vi "Mean between Cursers- Plugin Main.vi"(11 "Shared Data from EMA":T2={"Impulse Positions"=[], "Parameter Impuls Series"=[], "Data File"={"Data Channels"=[], "Sample Rate"=0, "Channel List"=[]}, "desacc "={"Threshold 1 [Acc]"=7000.0, "Threshold 2 [% of TH1]"=60, "tolerance"=3, "Search WD "=0.1, " always use TH2"=FALSE, "Range"=2.0, "Max time"=120.0, "Min time"=20.0, "Velocity Threshold"=150}, "Experiment Parameters 2"={"Subject"="", "Strain"="", "Rotation plane"="", "Experimenter"="", "Trial"=0.0, "Time"=0.0}} {"Parameter Impuls Series"."Gain" format="%.1f"; "Parameter Impuls Series"."Offset" format="%.1f"}) -> (3 "Shared Data from EMA 2":T2={"Impulse Positions"=[], "Parameter Impuls Series"=[], "Data File"={"Data Channels"=[], "Sample Rate"=0, "Channel List"=[]}, "desacc "={"Threshold 1 [Acc]"=7000.0, "Threshold 2 [% of TH1]"=60, "tolerance"=3, "Search WD "=0.1, " always use TH2"=FALSE, "Range"=2.0, "Max time"=120.0, "Min time"=20.0, "Velocity Threshold"=150}, "Experiment Parameters 2"={"Subject"="", "Strain"="", "Rotation plane"="", "Experimenter"="", "Trial"=0.0, "Time"=0.0}} {"Parameter Impuls Series"."Gain" format="%.1f"; "Parameter Impuls Series"."Offset" format="%.1f"})   [LabVIEW 2013]
uses:
  Plugin Shared Data.ctl
  core/type-defs/TD_Impulse Parameter.ctl
  res/controls/impuls graph/impuls graph.xctl
  <vilib>/Analysis/baseanly.llb/Mean (DBL).vi
  comm/impulse/impulse functions.lvlib
  <vilib>/Analysis/NI_AALBase.lvlib
  <vilib>/ptbypt/NI_PtbyPt.lvlib
  core/core.lvlib
  plugin data.lvlib
panel:
  out "Waveform Graph":dbl[][](graph)
  out "Impulse Plot":T1(xcontrol)
  in  "Delete trace":bool
  in  "Button toClipboard":bool
  in  "Button Save":bool
  in  "Table":string[][](table)
  out "Mean 1":dbl format="%#.3f"
  out "Mean 2":dbl format="%#.3f"
  out "Mean 2 SD":dbl format="%#.3f"
  in  "Button Calculate":bool
  out "Mean 1 SD":dbl format="%#.3f"
  in  "Parameter Impuls Series":T3=[{"Color"=4652800, "Visible"=TRUE, "Channel"=5, "Invert"=FALSE, "Desaccade"=FALSE, "Offset"=0.0, "Gain"=1.0}, {"Color"=16860, "Visible"=TRUE, "Channel"=13, "Invert"=FALSE, "Desaccade"=FALSE, "Offset"=0.0, "Gain"=1.0}, {"Color"=16711680, "Visible"=TRUE, "Channel"=21, "Invert"=FALSE, "Desaccade"=FALSE, "Offset"=0.0, "Gain"=1.0}] {"Gain" format="%.1f"; "Offset" format="%.1f"}
  in  "Impulse Direction":bool
  in  "Mean and STD":bool
  in  "Delete trace 2":bool
  in  "Stop Button":bool
  # "Offset         Gain    Inv                    Channel                         Col   Vis   Sac"
  # "Pos"
  # "Neg"
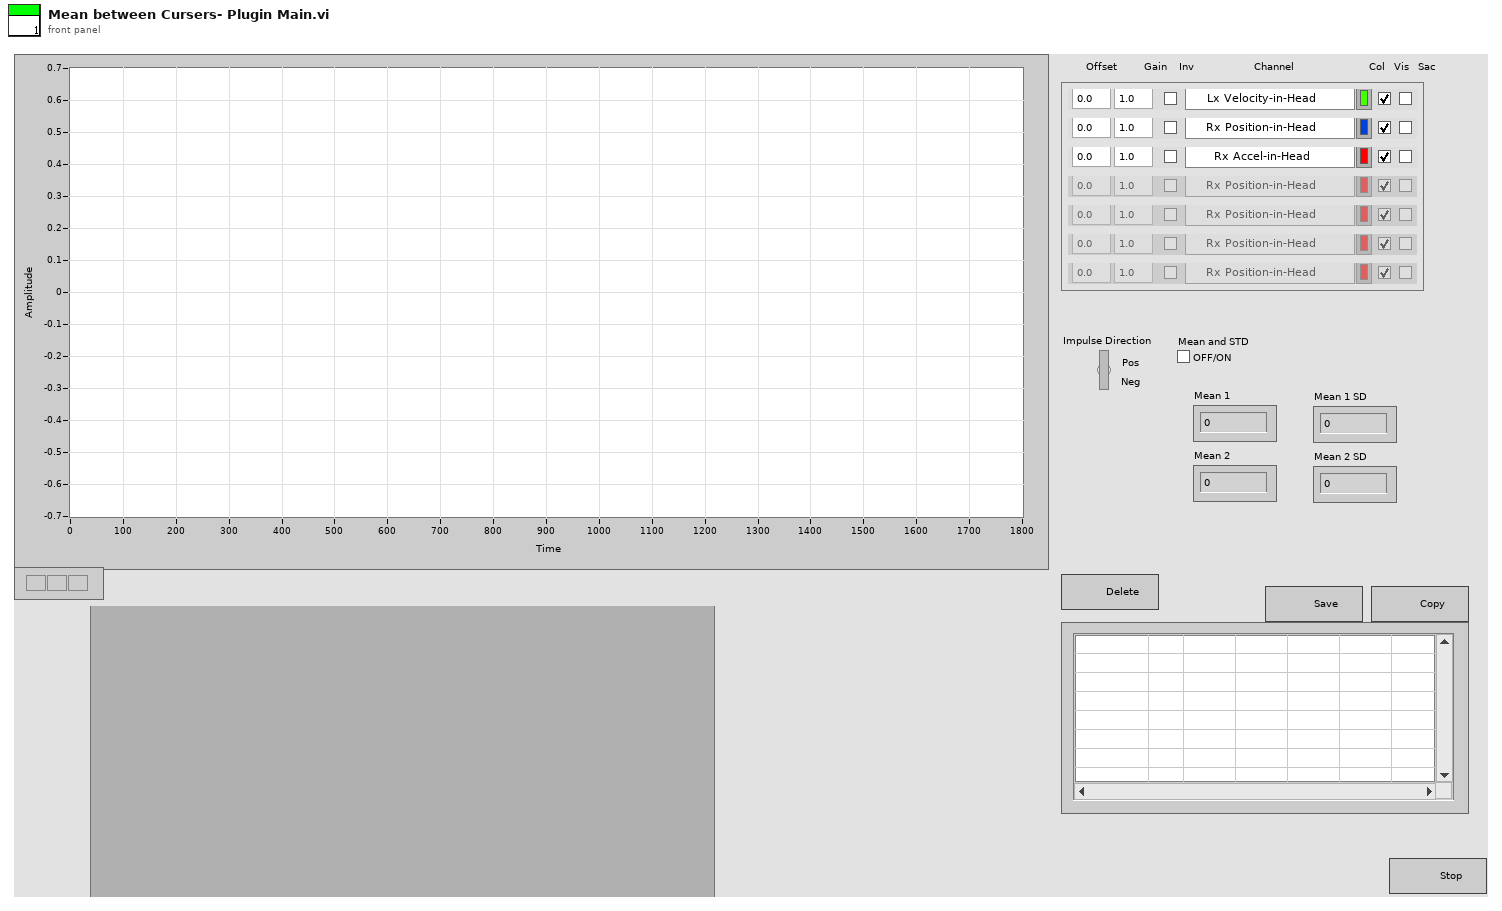
[diagram p1: front panel]
types:
  T1 = cluster{"Data":dbl[][], "Colour":u32, "Channel Name":string, "Sample Rate":dbl, "Visible":bool}[]
  T2 = typedef "plugin data.lvlib/Plugin Shared Data.ctl" = cluster{"Impulse Positions":cluster{"Start":i32, "End":i32, "Impulse Plane":enum16{"Other", "Yaw", "Pitch", "Roll", "LARP", "RALP"}, "Impulse Direction +ve?":bool, "Time offset":i32, "Amplitude offset":dbl}[], "Parameter Impuls Series":T3, "Data File":cluster{"Data Channels":dbl[][], "Sample Rate":i32, "Channel List":string[]}, "desacc ":cluster{"Threshold 1 [Acc]":dbl, "Threshold 2 [% of TH1]":i32, "tolerance":i32, "Search WD ":dbl, " always use TH2":bool, "Range":dbl, "Max time":dbl, "Min time":dbl, "Velocity Threshold":i32}, "Experiment Parameters 2":cluster{"Subject":string, "Strain":string, "Rotation plane":string, "Experimenter":string, "Trial":dbl, "Time":dbl}}
  T3 = typedef "core.lvlib/TD_Impulse Parameter.ctl" = cluster{"Color":u32, "Visible":bool, "Channel":u16, "Invert":bool, "Desaccade":bool, "Offset":dbl, "Gain":dbl}[]
  T4 = cluster{"Example Data":bool, "Impuls Data":cluster{"Data":dbl[][], "Colour":u32, "Channel Name":string, "Sample Rate":dbl, "Visible":bool}[], "K":dbl[], "cum pos data":dbl[][]}
  T5 = enum16{"Other", "Yaw", "Pitch", "Roll", "LARP", "RALP"}
  T6 = cluster{"Data Channels":dbl[][], "Sample Rate":i32, "Channel List":string[]}
  T7 = cluster{"Start":i32, "End":i32, "Impulse Plane":enum16{"Other", "Yaw", "Pitch", "Roll", "LARP", "RALP"}, "Impulse Direction +ve?":bool, "Time offset":i32, "Amplitude offset":dbl}[]
  T8 = cluster{"Threshold 1 [Acc]":dbl, "Threshold 2 [% of TH1]":i32, "tolerance":i32, "Search WD ":dbl, " always use TH2":bool, "Range":dbl, "Max time":dbl, "Min time":dbl, "Velocity Threshold":i32}
  T9 = typedef "LVCursorListTypeDef.ctl" = cluster{"Name":string, "Color":u32, "Style":u8, "Point Style":u8, "Name Visible":bool, "Allow Drag":bool, "Cursor Mode":u32, "Plot":i32, "Index":i32, "Position":cluster{"X":dbl, "Y":dbl}, "X Scale":u32, "Y Scale":u32, "Watch Plots":i32[], "Watch All Plots":bool, "Plot Area":i32, "Label Offset":cluster{"X":dbl, "Y":dbl}}[]
  T10 = cluster{"Name":string, "Color":u32, "Style":u8, "Point Style":u8, "Name Visible":bool, "Allow Drag":bool, "Cursor Mode":u32, "Plot":i32, "Index":i32, "Position":cluster{"X":dbl, "Y":dbl}, "X Scale":u32, "Y Scale":u32, "Watch Plots":i32[], "Watch All Plots":bool, "Plot Area":i32, "Label Offset":cluster{"X":dbl, "Y":dbl}}
  T11 = cluster{"Data":dbl[][], "Colour":u32, "Channel Name":string, "Sample Rate":dbl, "Visible":bool}
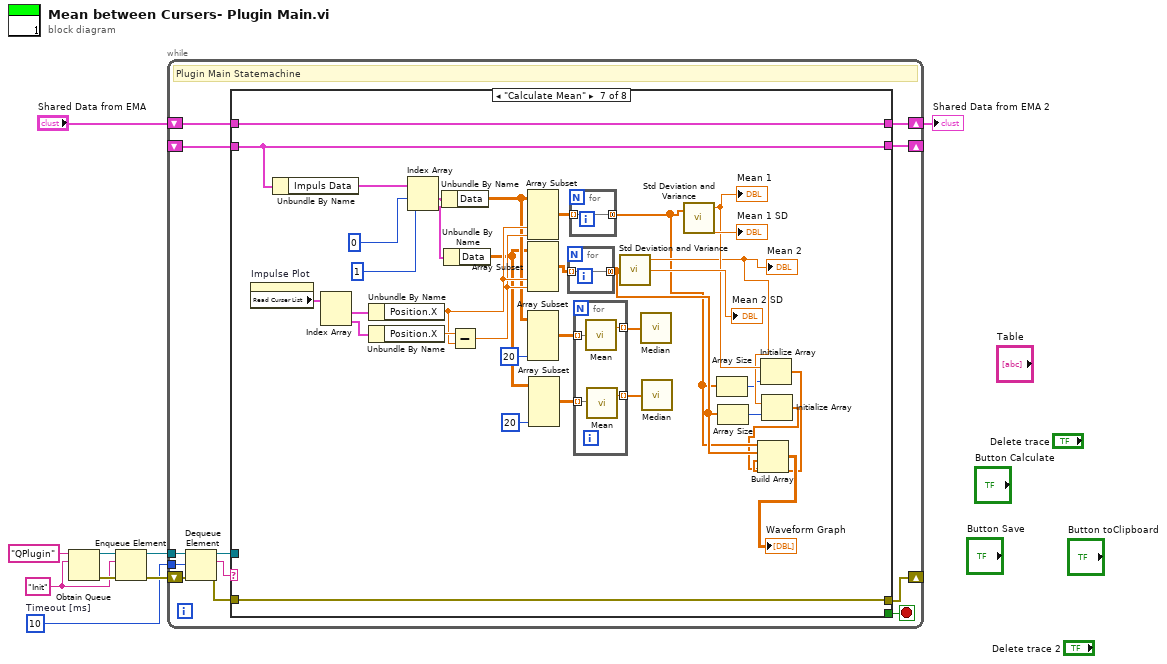
[diagram p0: block diagram]
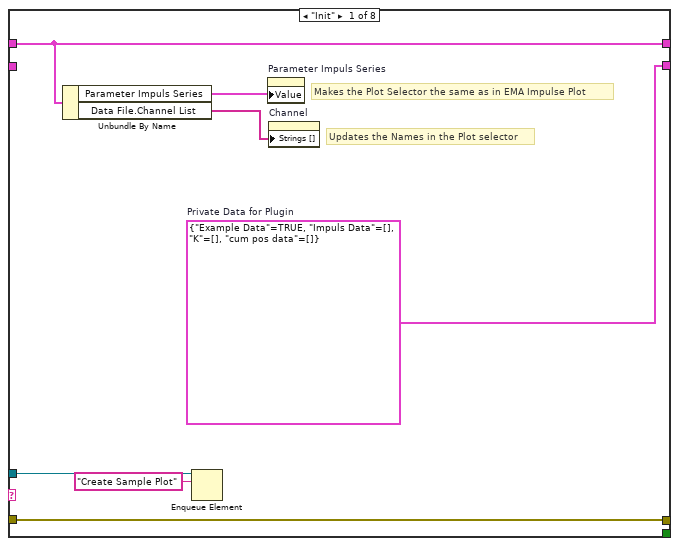
[diagram p2: hidden frame]
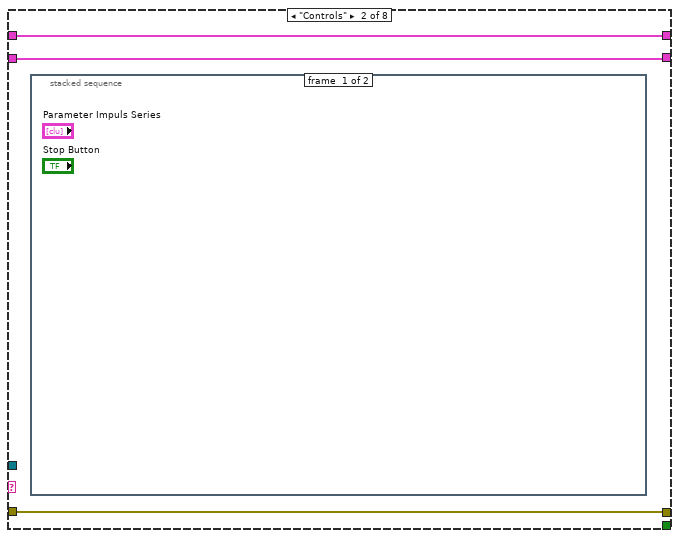
[diagram p3: hidden frame]
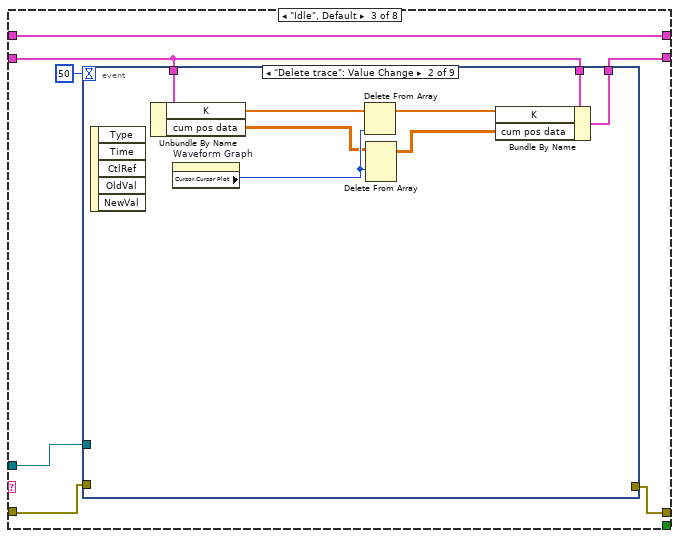
[diagram p5: hidden frame]
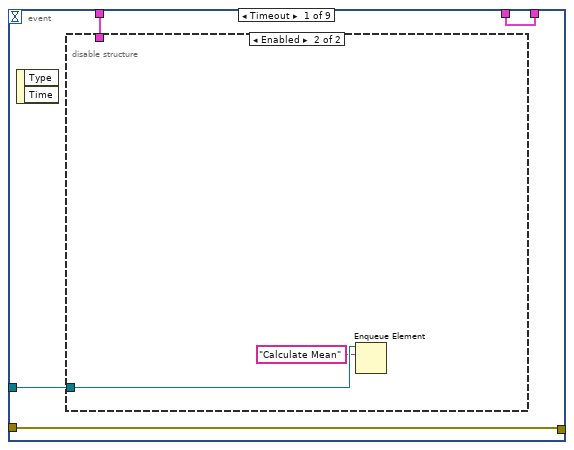
[diagram p6: hidden frame]
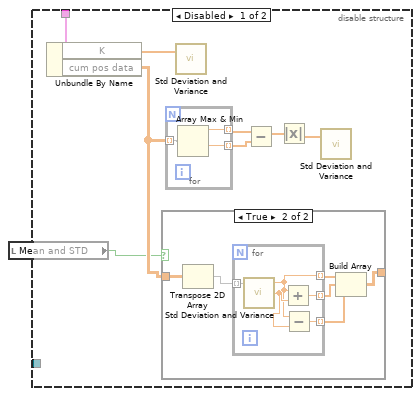
[diagram p7: hidden frame]
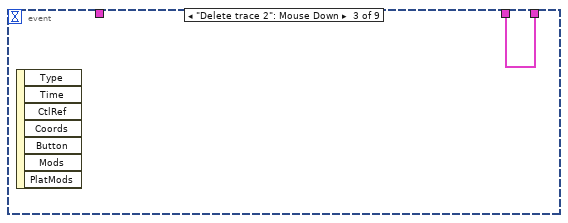
[diagram p9: hidden frame]
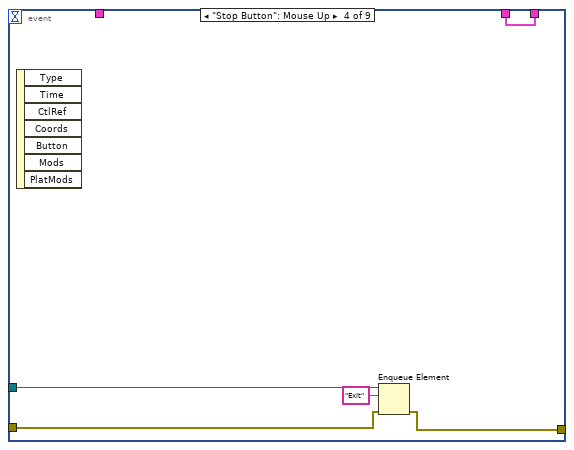
[diagram p10: hidden frame]
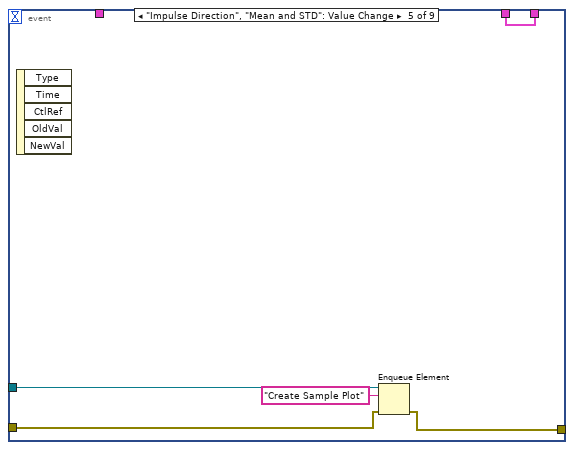
[diagram p11: hidden frame]
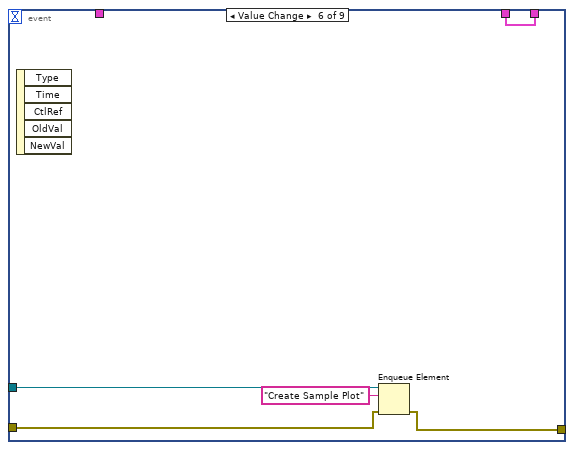
[diagram p12: hidden frame]
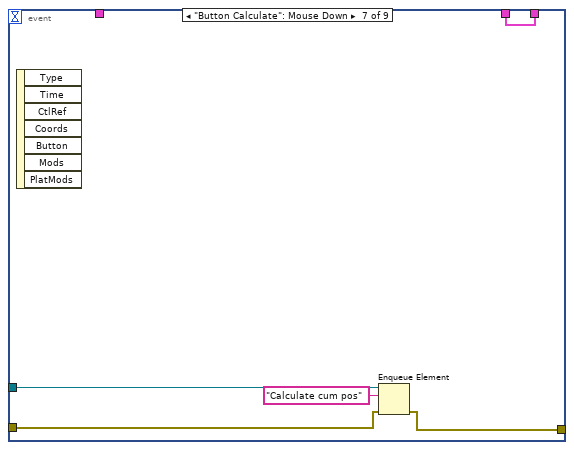
[diagram p13: hidden frame]
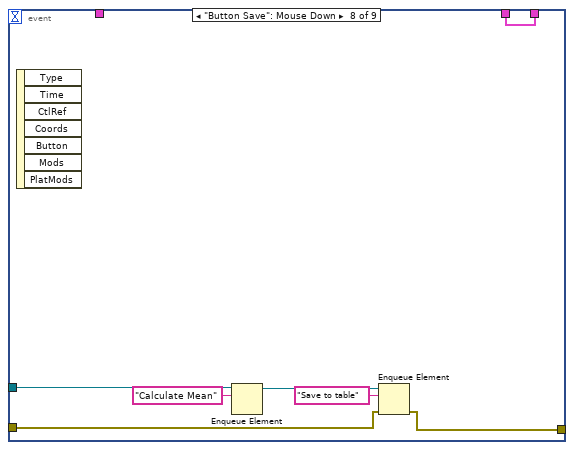
[diagram p14: hidden frame]
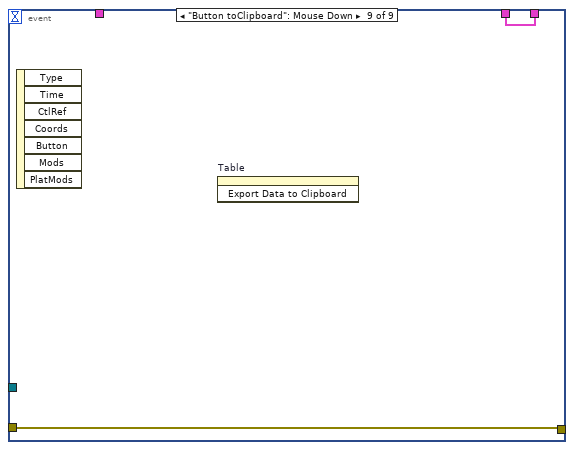
[diagram p15: hidden frame]
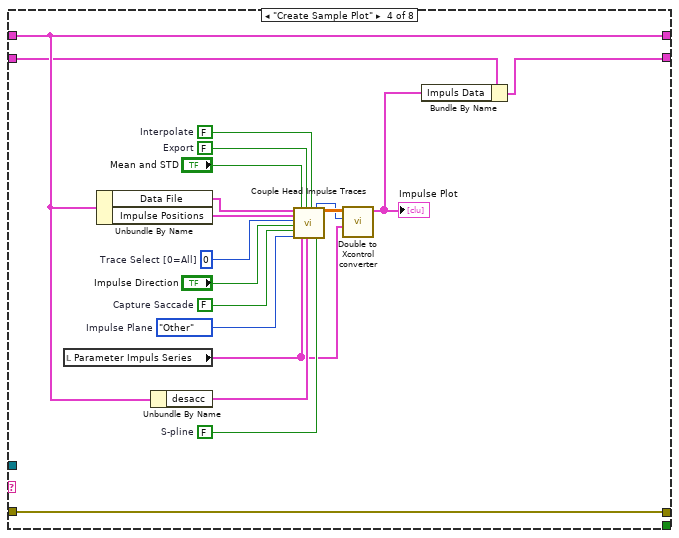
[diagram p16: hidden frame]
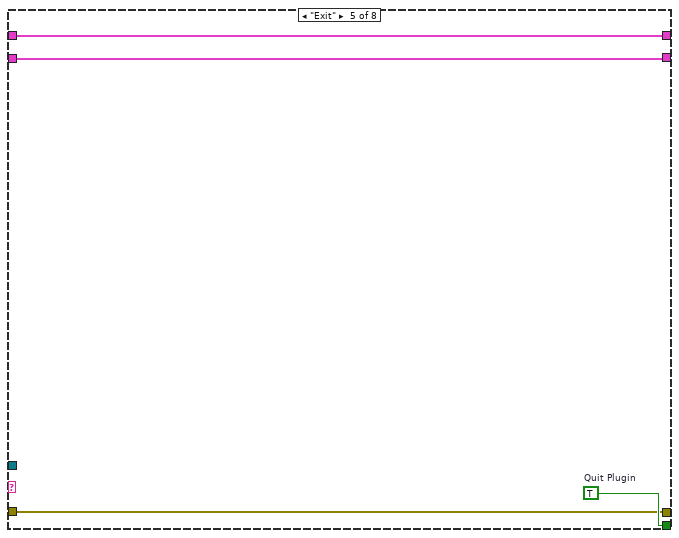
[diagram p17: hidden frame]
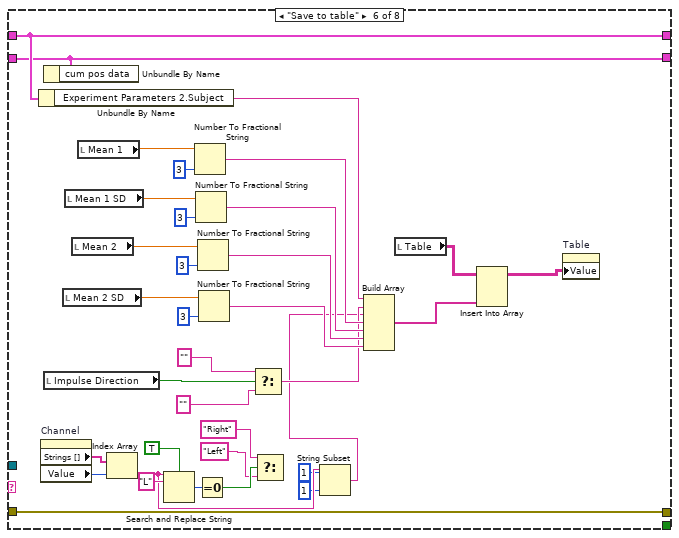
[diagram p18: hidden frame]
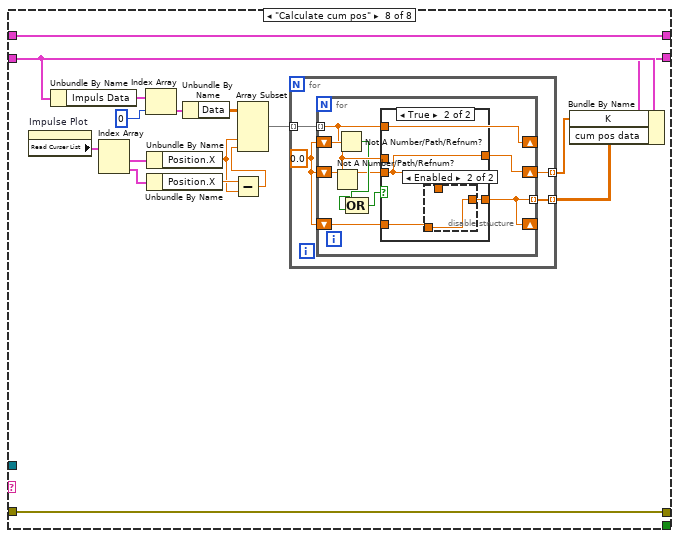
[diagram p19: hidden frame]
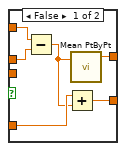
[diagram p20: hidden frame]
diagram:
  w3 = 10  # Timeout [ms]
  w7 = "Init"
  n1 = Obtain Queue(name (unnamed)="QPlugin", element data type=w7) -> (queue out=w8:refnum<queue>, error out=w9:errorcluster)  [unwired: 3 in, 1 out]
  n2 = Enqueue Element(queue=w8, element=w7, error in (no error)=w9) -> (queue out=w5:refnum<queue>, error out=w4:errorcluster)  [unwired: 1 in, 1 out]
  n3 = while {
    tunnel: w5 -> [w20]
    tunnel: w3 -> [w18]
    shift-right: [w14] -> _
    shift-left: w4 -> [w19]
    shift-right: [w13] -> _
    shift-left: _ -> [w12]
    shift-right: [w10] -> w1
    shift-left: "Shared Data from EMA" -> [w11]
    stop <- w21 stop-if-true
    # "Plugin Main Statemachine"
    n4 = Dequeue Element(queue=w20, timeout in ms (-1)=w18, error in (no error)=w19) -> (queue out=w17:refnum<queue>, element=w16:string, error out=w15:errorcluster)  [unwired: 1 out]
    n5 = case shown="\"Calculate Mean\"" w16 {
      tunnel: [_ _ _ _ w133 _ _ _] -> w21
      tunnel: w17 -> [w26 _ w37 _ _ _ _ _]
      tunnel: w15 -> [w27 w29 w36 w129 w132 w168 w203 w226]
      tunnel: [w27 w29 w35 w129 w132 w168 w203 w226] -> w14
      tunnel: [w28 w30 w32 w112 w131 w138 w201 w212] -> w13
      tunnel: w12 -> [_ w30 w33 w113 w131 w138 w201 w213]
      tunnel: w11 -> [w24 w31 w38 w119 w130 w167 w202 w225]
      tunnel: [w24 w31 w38 w119 w130 w167 w202 w225] -> w10
      frame "Init" {
        w28 = T4 {"Example Data"=TRUE, "Impuls Data"=[], "K"=[], "cum pos data"=[]}  # Private Data for Plugin
        # "Makes the Plot Selector the same as in EMA Impulse Plot"
        # "Updates the Names in the Plot selector"
        n6 = Unbundle By Name(w24) -> ("Parameter Impuls Series"=w23:T3, "Data File.Channel List"=w22:string[])
        n7 = Enqueue Element(queue=w26, element="Create Sample Plot") -> ()  [unwired: 2 in, 3 out]
        n8 = property on="Parameter Impuls Series" class="Arr (strict)"("Value"=w23) -> ()  [unwired: 2 in, 2 out]
        n9 = property on="Channel" class="Ring (strict)"("Strings []"=w22) -> ()  [unwired: 2 in, 2 out]
      }
      frame "Controls" {
        n10 = stacked-sequence {
          frame #0 {
          }
          frame #1 {
          }
        }
      }
      frame "Idle", Default {
        n11 = event shown="[1] \"Delete trace\": Value Change" {
          selector: _ -> [_ _ _ _ _ _ _ _ _]
          dyn-events: _ -> [_ _ _ _ _ _ _ _ _]
          timeout: 50 -> [_ _ _ _ _ _ _ _ _]
          tunnel: w37 -> [w39 _ _ w86 w91 w96 w101 w105 _]
          tunnel: w36 -> [w42 _ _ w84 w89 w94 w99 w107 w110]
          tunnel: [w42 _ _ w83 w88 w93 w98 w106 w110] -> w35
          tunnel: w33 -> [w41 w80 _ _ _ _ _ _ _]
          tunnel: w33 -> [w40 w78 w81 w82 w87 w92 w97 w102 w109]
          tunnel: [w40 w75 w81 w82 w87 w92 w97 w102 w109] -> w32
          event Timeout {
            n12 = event-data() -> ()  [unwired: 1 in, 2 out]
            n13 = disable-structure shown="Enabled" {
              disable-tunnel: w41 -> [w55 _]
              disable-tunnel: w39 -> [_ w72]
              frame Disabled {
                n14 = local read "Mean and STD"() -> (w49:bool)
                n15 = Unbundle By Name(w55) -> ("K"=w43:dbl[], "cum pos data"=w51:dbl[][])
                n16 = case shown="True" w49 {
                  tunnel: w51 -> [w56 w62]
                  tunnel: [w56 w59] -> w50
                  frame False {
                  }
                  frame True {
                    n17 = Transpose 2D Array(2D array=w62) -> (transposed array=w61:dbl[][])
                    n18 = for {
                      tunnel: w61 -> [w67] mode=indexing
                      tunnel: [w63] -> w60 mode=indexing
                      tunnel: [w65] -> w58 mode=indexing
                      tunnel: [w64] -> w57 mode=indexing
                      n19 = call <vilib>:"Std Deviation and Variance.vi"("X"=w67) -> ("mean"=w63:dbl, "standard deviation"=w66:dbl)  [unwired: 1 in, 1 out]
                      n20 = Add(x=w63, y=w66) -> (x+y=w65:dbl)
                      n21 = Subtract(x=w63, y=w66) -> (x-y=w64:dbl)
                    }
                    n22 = Build Array(w60, w58, w57) -> (w59:dbl[][])
                  }
                }
                n23 = for {
                  tunnel: w51 -> [w70] mode=indexing
                  tunnel: [w69] -> w54 mode=indexing
                  tunnel: [w68] -> w53 mode=indexing
                  n24 = Array Max & Min(array=w70) -> (max value=w69:dbl, min value=w68:dbl)  [unwired: 2 out]
                }
                n25 = call <vilib>:"Std Deviation and Variance.vi"("X"=w43) -> ("mean"=w44:dbl, "standard deviation"=w45:dbl)  [unwired: 1 in, 1 out]
                n26 = Subtract(x=w54, y=w53) -> (x-y=w52:dbl[])
                n27 = Absolute Value(x=w52) -> (abs(x)=w48:dbl[])
                n28 = call <vilib>:"Std Deviation and Variance.vi"("X"=w48) -> ("mean"=w47:dbl, "standard deviation"=w46:dbl)  [unwired: 1 in, 1 out]
              }
              frame Enabled {
                n29 = Enqueue Element(queue=w72, element="Calculate Mean") -> ()  [unwired: 2 in, 3 out]
              }
            }
          }
          event "Delete trace": Value Change {
            n30 = event-data() -> ()  [unwired: 1 in, 5 out]
            n31 = Unbundle By Name(w80) -> ("K"=w79:dbl[], "cum pos data"=w73:dbl[][])
            n32 = property on="Waveform Graph" class="WFGraph (strict)"() -> ("Cursor.Cursor Plot"=w74:i32)  [unwired: 2 in, 2 out]
            n33 = Delete From Array(array=w79, index=w74) -> (array with subset deleted=w77:dbl[])  [unwired: 1 in, 1 out]
            n34 = Delete From Array(array=w73, index (row)=w74) -> (array with subset deleted=w76:dbl[][])  [unwired: 2 in, 1 out]
            n35 = Bundle By Name(cluster=w78, "K"=w77, "cum pos data"=w76) -> (w75:T4)
          }
          event "Delete trace 2": Mouse Down {
            n36 = event-data() -> ()  [unwired: 1 in, 7 out]
          }
          event "Stop Button": Mouse Up {
            n37 = event-data() -> ()  [unwired: 1 in, 7 out]
            n38 = Enqueue Element(queue=w86, element="Exit", error in (no error)=w84) -> (error out=w83:errorcluster)  [unwired: 1 in, 2 out]
          }
          event "Impulse Direction", "Mean and STD": Value Change {
            n39 = event-data() -> ()  [unwired: 1 in, 5 out]
            n40 = Enqueue Element(queue=w91, element="Create Sample Plot", error in (no error)=w89) -> (error out=w88:errorcluster)  [unwired: 1 in, 2 out]
          }
          event Value Change {
            n41 = event-data() -> ()  [unwired: 1 in, 5 out]
            n42 = Enqueue Element(queue=w96, element="Create Sample Plot", error in (no error)=w94) -> (error out=w93:errorcluster)  [unwired: 1 in, 2 out]
          }
          event "Button Calculate": Mouse Down {
            n43 = event-data() -> ()  [unwired: 1 in, 7 out]
            n44 = Enqueue Element(queue=w101, element="Calculate cum pos", error in (no error)=w99) -> (error out=w98:errorcluster)  [unwired: 1 in, 2 out]
          }
          event "Button Save": Mouse Down {
            n45 = event-data() -> ()  [unwired: 1 in, 7 out]
            n46 = Enqueue Element(queue=w105, element="Calculate Mean") -> (queue out=w104:refnum<queue>)  [unwired: 2 in, 2 out]
            n47 = Enqueue Element(queue=w104, element="Save to table", error in (no error)=w107) -> (error out=w106:errorcluster)  [unwired: 1 in, 2 out]
          }
          event "Button toClipboard": Mouse Down {
            n48 = event-data() -> ()  [unwired: 1 in, 7 out]
            n49 = invoke on="Table" class="Tbl (strict)" method="Export Data to Clipboard"() -> ()  [unwired: 3 in, 3 out]
          }
        }
      }
      frame "Create Sample Plot" {
        w117 = FALSE  # S-pline
        w120 = FALSE  # Interpolate
        w121 = FALSE  # Export
        w123 = T5."Other"  # Impulse Plane
        w124 = FALSE  # Capture Saccade
        w126 = 0  # Trace Select [0=All]
        n50 = local read "Parameter Impuls Series"() -> (w114:T3)
        n51 = Unbundle By Name(w119) -> ("Data File"=w127:T6, "Impulse Positions"=w128:T7)
        n52 = Unbundle By Name(w119) -> ("desacc"=w118:T8)
        n53 = call "Couple Head Impulse Traces.vi"("Data Input"=w127, "Impulse Positions"=w128, "Trace Select"=w126, "Impulse Direction +ve?"="Impulse Direction", "Capture Saccade"=w124, "Impulse Plane"=w123, "Mean and STD"="Mean and STD", "Plot Selection 2"=w114, "Export"=w121, "desacc"=w118, "Interpolate"=w120, "S-pline"=w117) -> ("No Impulses"=w115:i32, "Impulses"=w116:dbl[][])  [unwired: 4 in, 2 out]
        n54 = call "Double to Xcontrol converter.vi"("Parameter Impuls Series"=w114, "No Impulses"=w115, "Impulses"=w116) -> ("Array"=w111:T1)  [unwired: 8 in]
        "Impulse Plot" <- w111
        n55 = Bundle By Name(cluster=w113, "Impuls Data"=w111) -> (w112:T4)
      }
      frame "Exit" {
        w133 = TRUE  # Quit Plugin
      }
      frame "Save to table" {
        n56 = Unbundle By Name(w167) -> ("Experiment Parameters 2.Subject"=w165:string)
        n57 = property on="Channel" class="Ring (strict)"() -> ("Strings []"=w146:string[], "Value"=w145:u16)  [unwired: 2 in, 2 out]
        n58 = Unbundle By Name(w138) -> ()  [unwired: 1 out]
        n59 = local read "Impulse Direction"() -> (w150:bool)
        n60 = local read "Mean 2 SD"() -> (w155:dbl)
        n61 = local read "Mean 1 SD"() -> (w157:dbl)
        n62 = local read "Mean 2"() -> (w156:dbl)
        n63 = local read "Mean 1"() -> (w164:dbl)
        n64 = Index Array(array=w146, index=w145) -> (element=w137:string)
        n65 = Search and Replace String(case sensitive?=TRUE ("ignore case? (F)"), input string=w137, search string="L") -> (number of replacements=w142:i32)  [unwired: 5 in, 3 out]
        n66 = Number To Fractional String(number=w164, precision (6)=i16 3) -> (F-format string=w154:string)  [unwired: 2 in]
        n67 = Number To Fractional String(number=w157, precision (6)=i16 3) -> (F-format string=w153:string)  [unwired: 2 in]
        n68 = Equal To 0?(x=w142) -> (x = 0?=w141:bool)
        n69 = Number To Fractional String(number=w156, precision (6)=i16 3) -> (F-format string=w152:string)  [unwired: 2 in]
        n70 = Number To Fractional String(number=w155, precision (6)=i16 3) -> (F-format string=w151:string)  [unwired: 2 in]
        n71 = Select(t="", s=w150, f="") -> (s? t:f=w149:string)
        n72 = Select(t="Right", s=w141, f="Left") -> ()  [unwired: 1 out]
        n73 = String Subset(string=w137, offset (0)=1, length (rest)=1 ("length (rest)")) -> (substring=w135:string)
        n74 = Build Array(w165, w149, w135, w154, w153, w152, w151) -> (w162:string[])
        n75 = local read "Table"() -> (w166:string[][])
        n76 = Insert Into Array(array=w166, new element=w162) -> (w161:string[][])  [unwired: 2 in]
        n77 = property on="Table" class="Tbl (strict)"("Value"=w161) -> ()  [unwired: 2 in, 2 out]
      }
      frame "Calculate Mean" {
        n78 = property on="Impulse Plot" class="impuls graph (strict)"() -> ("Read Curser List"=w197:T9)  [unwired: 2 in, 2 out]
        n79 = Unbundle By Name(w201) -> ("Impuls Data"=w200:T1)
        n80 = Index Array(array=w197) -> (element #1=w196:T10, element #2=w195:T10)  [unwired: 2 in]
        n81 = Unbundle By Name(w196) -> ("Position.X"=w191:dbl)
        n82 = Unbundle By Name(w195) -> ("Position.X"=w194:dbl)
        n83 = Index Array(array=w200, index #1=0 ("index"), index #2=1 ("index")) -> (element #1=w198:T11, element #2=w192:T11)
        n84 = Unbundle By Name(w198) -> ("Data"=w189:dbl[][])
        n85 = Unbundle By Name(w192) -> ("Data"=w188:dbl[][])
        n86 = Subtract(x=w194, y=w191) -> (x-y=w190:dbl)
        n87 = Array Subset(array=w189, index (col)=w191, length (col)=w190) -> (w179:dbl[][])  [unwired: 2 in]
        n88 = Array Subset(array=w188, index (col)=w191, length (col)=w190) -> (w178:dbl[][])  [unwired: 2 in]
        n89 = Array Subset(array=w189, length (col)=20 ("length")) -> (w185:dbl[][])  [unwired: 3 in]
        n90 = Array Subset(array=w188, length (col)=20 ("length")) -> (w184:dbl[][])  [unwired: 3 in]
        n91 = for {
          tunnel: w178 -> [w204] mode=indexing
          tunnel: [w204] -> w174 mode=concatenating
        }
        n92 = for {
          tunnel: w179 -> [w205] mode=indexing
          tunnel: [w205] -> w171 mode=concatenating
        }
        n93 = for {
          tunnel: w185 -> [w209] mode=indexing
          tunnel: w184 -> [w208] mode=indexing
          tunnel: [w207] -> w182 mode=indexing
          tunnel: [w206] -> w183 mode=indexing
          n94 = call-poly <vilib>:"Mean.vi"("X"=w209) -> ("mean"=w206:dbl)  [unwired: 1 out]
          n95 = call-poly <vilib>:"Mean.vi"("X"=w208) -> ("mean"=w207:dbl)  [unwired: 1 out]
        }
        n96 = call <vilib>:"Std Deviation and Variance.vi"("X"=w174) -> ("mean"=w175:dbl, "standard deviation"=→"Mean 2 SD":dbl)  [unwired: 1 in, 1 out]
        "Mean 2" <- w175
        n97 = call <vilib>:"Median.vi"("X"=w183) -> ()  [unwired: 2 out]
        n98 = call <vilib>:"Median.vi"("X"=w182) -> ()  [unwired: 2 out]
        n99 = call <vilib>:"Std Deviation and Variance.vi"("X"=w171) -> ("mean"=w176:dbl, "standard deviation"=→"Mean 1 SD":dbl)  [unwired: 1 in, 1 out]
        "Mean 1" <- w176
        n100 = Array Size(array=w171) -> (size(s)=w172:i32)
        n101 = Array Size(array=w174) -> (size(s)=w173:i32)
        n102 = Initialize Array(w176, w172) -> (w170:dbl[])
        n103 = Initialize Array(w175, w173) -> (w169:dbl[])
        n104 = Build Array(w171, w174, w170, w169) -> (→"Waveform Graph":dbl[][])
      }
      frame "Calculate cum pos" {
        n105 = property on="Impulse Plot" class="impuls graph (strict)"() -> ("Read Curser List"=w221:T9)  [unwired: 2 in, 2 out]
        n106 = Unbundle By Name(w213) -> ("Impuls Data"=w224:T1)
        n107 = Index Array(array=w221) -> (element #1=w220:T10, element #2=w219:T10)  [unwired: 2 in]
        n108 = Index Array(array=w224, index=0) -> (element=w222:T11)
        n109 = Unbundle By Name(w220) -> ("Position.X"=w216:dbl)
        n110 = Unbundle By Name(w219) -> ("Position.X"=w217:dbl)
        n111 = Unbundle By Name(w222) -> ("Data"=w218:dbl[][])
        n112 = Subtract(x=w217, y=w216) -> (x-y=w215:dbl)
        n113 = Array Subset(array=w218, index (col)=w216, length (col)=w215) -> (w214:dbl[][])  [unwired: 2 in]
        n114 = for {
          tunnel: w214 -> [w230] mode=indexing
          tunnel: [w229] -> w210 mode=indexing
          tunnel: [w227] -> w211 mode=indexing
          w228 = 0.0
          n115 = for {
            tunnel: w230 -> [w238] mode=indexing
            shift-right: [w238] -> _
            shift-left: w228 -> [w239]
            tunnel: [w233] -> w229 mode=indexing
            shift-right: [w233] -> _
            shift-left: w228 -> [w234]
            shift-right: [w232] -> w227
            shift-left: w228 -> [w231]
            n116 = Not A Number/Path/Refnum?(number/path/refnum=w239) -> (NaN/Path/Refnum?=w236:bool)
            n117 = Not A Number/Path/Refnum?(number/path/refnum=w238) -> (NaN/Path/Refnum?=w237:bool)
            n118 = Compound Arithmetic op=OR(w237, w236) -> (w235:bool)
            n119 = case shown="True" w235 {
              tunnel: w238 -> [w245 _]
              tunnel: w239 -> [w244 _]
              tunnel: [w243 w247] -> w233
              tunnel: w234 -> [w242 w248]
              tunnel: [w240 w246] -> w232
              tunnel: w231 -> [_ w246]
              frame False {
                n120 = Subtract(x=w245, y=w244) -> (x-y=w241:dbl)
                n121 = Add(x=w242, y=w241) -> (x+y=w243:dbl)
                n122 = call <vilib>:"Mean PtByPt.vi"("x"=w241) -> ("mean"=w240:dbl)  [unwired: 3 in, 1 out]
              }
              frame True {
                n123 = disable-structure shown="Enabled" {
                  disable-tunnel: w248 -> [w251 w252]
                  disable-tunnel: [w250 w252] -> w247
                  disable-tunnel: w246 -> [w249 _]
                  frame Disabled {
                    n124 = Add(x=w251, y=w249) -> (x+y=w250:dbl)
                  }
                  frame Enabled {
                  }
                }
              }
            }
          }
        }
        n125 = Bundle By Name(cluster=w213, "K"=w211, "cum pos data"=w210) -> (w212:T4)
      }
    }
  }
  "Shared Data from EMA 2" <- w1
